vi "remap.vi"(3 "BLUE":u32, 4 "GREEN":u32, 5 "RED":u32) -> (0 "BLUE 2":u32, 1 "GREEN 2":u32, 2 "RED 2":u32)   [LabVIEW 2020]
panel:
  # "Από την συχνότητα στο RGB"
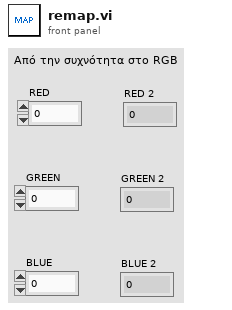
[diagram p1: front panel]
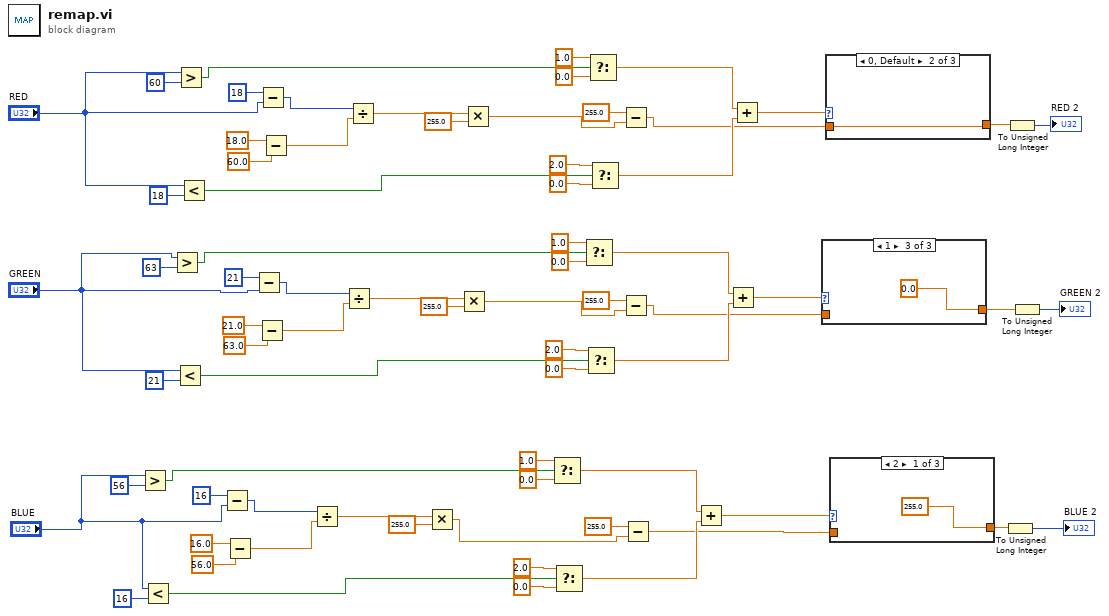
[diagram p0: block diagram]
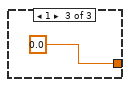
[diagram p3: hidden frame]
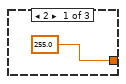
[diagram p4: hidden frame]
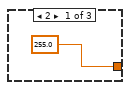
[diagram p6: hidden frame]
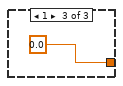
[diagram p7: hidden frame]
diagram:
  n1 = Greater?(x="BLUE", y=i64 56) -> (0:w25:bool)
  n2 = Less?(x="BLUE", y=i64 16) -> (x < y?=w20:bool)
  n3 = Greater?(x="GREEN", y=i64 63) -> (0:w44:bool)
  n4 = Less?(x="GREEN", y=i64 21) -> (x < y?=w39:bool)
  n5 = Greater?(x="RED", y=i64 60) -> (0:w62:bool)
  n6 = Less?(x="RED", y=i64 18) -> (x < y?=w57:bool)
  n7 = Subtract(x=i64 16, y="BLUE") -> (x-y=w29:i64)
  n8 = Subtract(x=16.0, y=56.0) -> (x-y=w28:dbl)
  n9 = Subtract(x=i64 21, y="GREEN") -> (x-y=w48:i64)
  n10 = Subtract(x=21.0, y=63.0) -> (x-y=w47:dbl)
  n11 = Subtract(x=i64 18, y="RED") -> (x-y=w66:i64)
  n12 = Subtract(x=18.0, y=60.0) -> (x-y=w65:dbl)
  n13 = Divide(x=w29, y=w28) -> (x/y=w27:dbl)
  n14 = Divide(x=w48, y=w47) -> (x/y=w46:dbl)
  n15 = Divide(x=w66, y=w65) -> (x/y=w64:dbl)
  n16 = Multiply(x=w27, y=255.0) -> (x*y=w7:dbl)
  n17 = Multiply(x=w46, y=255.0) -> (x*y=w8:dbl)
  n18 = Multiply(x=w64, y=255.0) -> (x*y=w14:dbl)
  n19 = Select(t=1.0, s=w25, f=0.0) -> (s? t:f=w19:dbl)
  n20 = Select(t=2.0, s=w20, f=0.0) -> (s? t:f=w18:dbl)
  n21 = Select(t=1.0, s=w44, f=0.0) -> (s? t:f=w38:dbl)
  n22 = Select(t=2.0, s=w39, f=0.0) -> (s? t:f=w37:dbl)
  n23 = Select(t=1.0, s=w62, f=0.0) -> (s? t:f=w56:dbl)
  n24 = Select(t=2.0, s=w57, f=0.0) -> (s? t:f=w55:dbl)
  n25 = Subtract(x=255.0, y=w14) -> (x-y=w13:dbl)
  n26 = Subtract(x=255.0, y=w8) -> (x-y=w11:dbl)
  n27 = Subtract(x=255.0, y=w7) -> (x-y=w12:dbl)
  n28 = Add(x=w19, y=w18) -> (x+y=w17:dbl)
  n29 = Add(x=w38, y=w37) -> (x+y=w36:dbl)
  n30 = Add(x=w56, y=w55) -> (x+y=w54:dbl)
  n31 = case shown="1" w36 {
    tunnel: [255.0 w74 0.0] -> w4
    tunnel: w11 -> [_ w74 _]
    frame 2 {
    }
    frame 0, Default {
    }
    frame 1 {
    }
  }
  n32 = case shown="0, Default" w54 {
    tunnel: [255.0 w77 0.0] -> w6
    tunnel: w13 -> [_ w77 _]
    frame 2 {
    }
    frame 0, Default {
    }
    frame 1 {
    }
  }
  n33 = case shown="2" w17 {
    tunnel: [255.0 w80 0.0] -> w3
    tunnel: w12 -> [_ w80 _]
    frame 2 {
    }
    frame 0, Default {
    }
    frame 1 {
    }
  }
  n34 = To Unsigned Long Integer(number=w3) -> (unsigned 32bit integer=→"BLUE 2":u32)
  n35 = To Unsigned Long Integer(number=w6) -> (unsigned 32bit integer=→"RED 2":u32)
  n36 = To Unsigned Long Integer(number=w4) -> (unsigned 32bit integer=→"GREEN 2":u32)
